vi "Configure Serial Bus (M1553 - Basic).vi"(0 "VISA resource name":refnum<visa-resource-name>, 1 "Source (0: Channel 1)":i32(ring) items=["Channel 1", "Channel 2", "Channel 3", "Channel 4"], 5 "Serial Bus Name (1: Serial Bus 1)":i32(ring)=1 items=["Serial Bus 1"=1, "Serial Bus 2"=2], 9 "Display Base (1: Hex)":i32(ring)=1 items=["Binary", "Hex"], 11 "error in (no error)":errorcluster) -> (4 "VISA resource name out":refnum<visa-resource-name>, 15 "error out":errorcluster)   [LabVIEW 2010, in "Agilent 2000 3000 X-Series.lvlib"]
doc: "Configures the basic settings of MIL- STD- 1553 bus."
uses:
  <instrlib>/Agilent 2000 3000 X-Series/Agilent 2000 3000 X-Series.lvlib
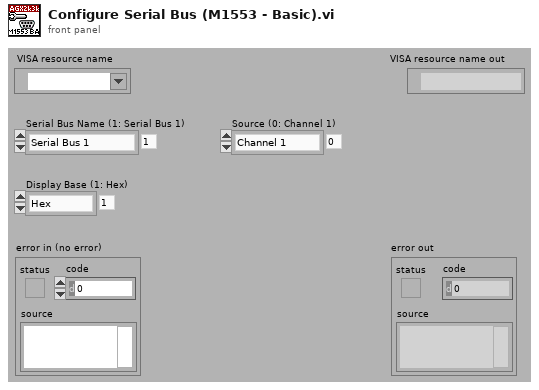
[diagram p1: front panel]
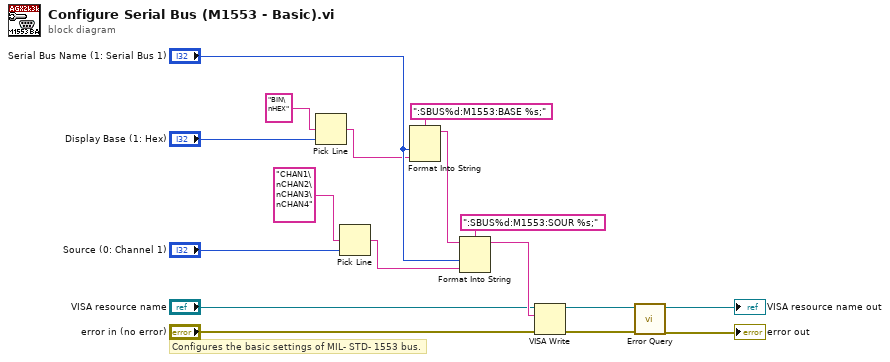
[diagram p0: block diagram]
diagram:
  # "Configures the basic settings of MIL- STD- 1553 bus."
  n1 = Pick Line(multi-line string="BIN\nHEX", line index="Display Base (1: Hex)") -> (output string=w13:string)  [unwired: 1 out]
  n2 = Pick Line(multi-line string="CHAN1\nCHAN2\nCHAN3\nCHAN4", line index="Source (0: Channel 1)") -> (output string=w8:string)  [unwired: 1 out]
  n3 = Format Into String(format string=":SBUS%d:M1553:BASE %s;", "Serial Bus Name (1: Serial Bus 1)", w13) -> (resulting string=w10:string)  [unwired: 2 in, 1 out]
  n4 = Format Into String(format string=":SBUS%d:M1553:SOUR %s;", initial string=w10, "Serial Bus Name (1: Serial Bus 1)", w8) -> (resulting string=w7:string)  [unwired: 1 in, 1 out]
  n5 = VISA Write(VISA resource name="VISA resource name", write buffer=w7, error in (no error)="error in (no error)") -> (VISA resource name out=w4:refnum<visa-resource-name>, error out=w3:errorcluster)  [unwired: 1 out]
  n6 = call <instrlib>:"Error Query.vi"("error in (no error)"=w3, "VISA resource name"=w4) -> ("error out"=→"error out":errorcluster, "VISA resource name out"=→"VISA resource name out":refnum<visa-resource-name>)  [unwired: 8 out]
